vi "Create Fast Draw Object.vi"(6 "Actual Transform In":T1, 8 "error in (no error)":errorcluster, 9 "Multiplot Representation In":T3, 10 "3D Bar.lvclass in":refnum<class "3D Bar.lvclass">, 11 "Plot Object In":refnum<vi>) -> (0 "error out":errorcluster, 1 "Multiplot Representation Out":T3, 2 "3D Bar.lvclass out":refnum<class "3D Bar.lvclass">, 3 "Plot Object Out":refnum<vi>, 4 "Actual Transform Out":T1)   [LabVIEW 2017, in "3D Bar.lvclass"]
uses:
  <vilib>/Math Plots/3D Math Plots/3D Bar/3D Bar/3D Bar.lvclass
  <vilib>/Math Plots/3D Math Plots/3D Plot/3D Plot/Typedef/Multiplot Representation.ctl
  <vilib>/Math Plots/3D Math Plots/3D Plot/3D Plot/Typedef/Plot Representation.ctl
  <vilib>/Math Plots/3D Math Plots/3D Plot/3D Plot/Typedef/Range Clusters.ctl
  <vilib>/Math Plots/3D Math Plots/3D Plot/3D Plot/Typedef/Mesh Data.ctl
  <vilib>/Math Plots/3D Math Plots/3D Plot/3D Plot/Typedef/Actual Transform.ctl
  <vilib>/Math Plots/3D Math Plots/3D Bar/3D Bar/3D Bar.lvclass/3D Bar.ctl
  <vilib>/Math Plots/3D Math Plots/3D Plot/3D Plot/3D Plot.lvclass
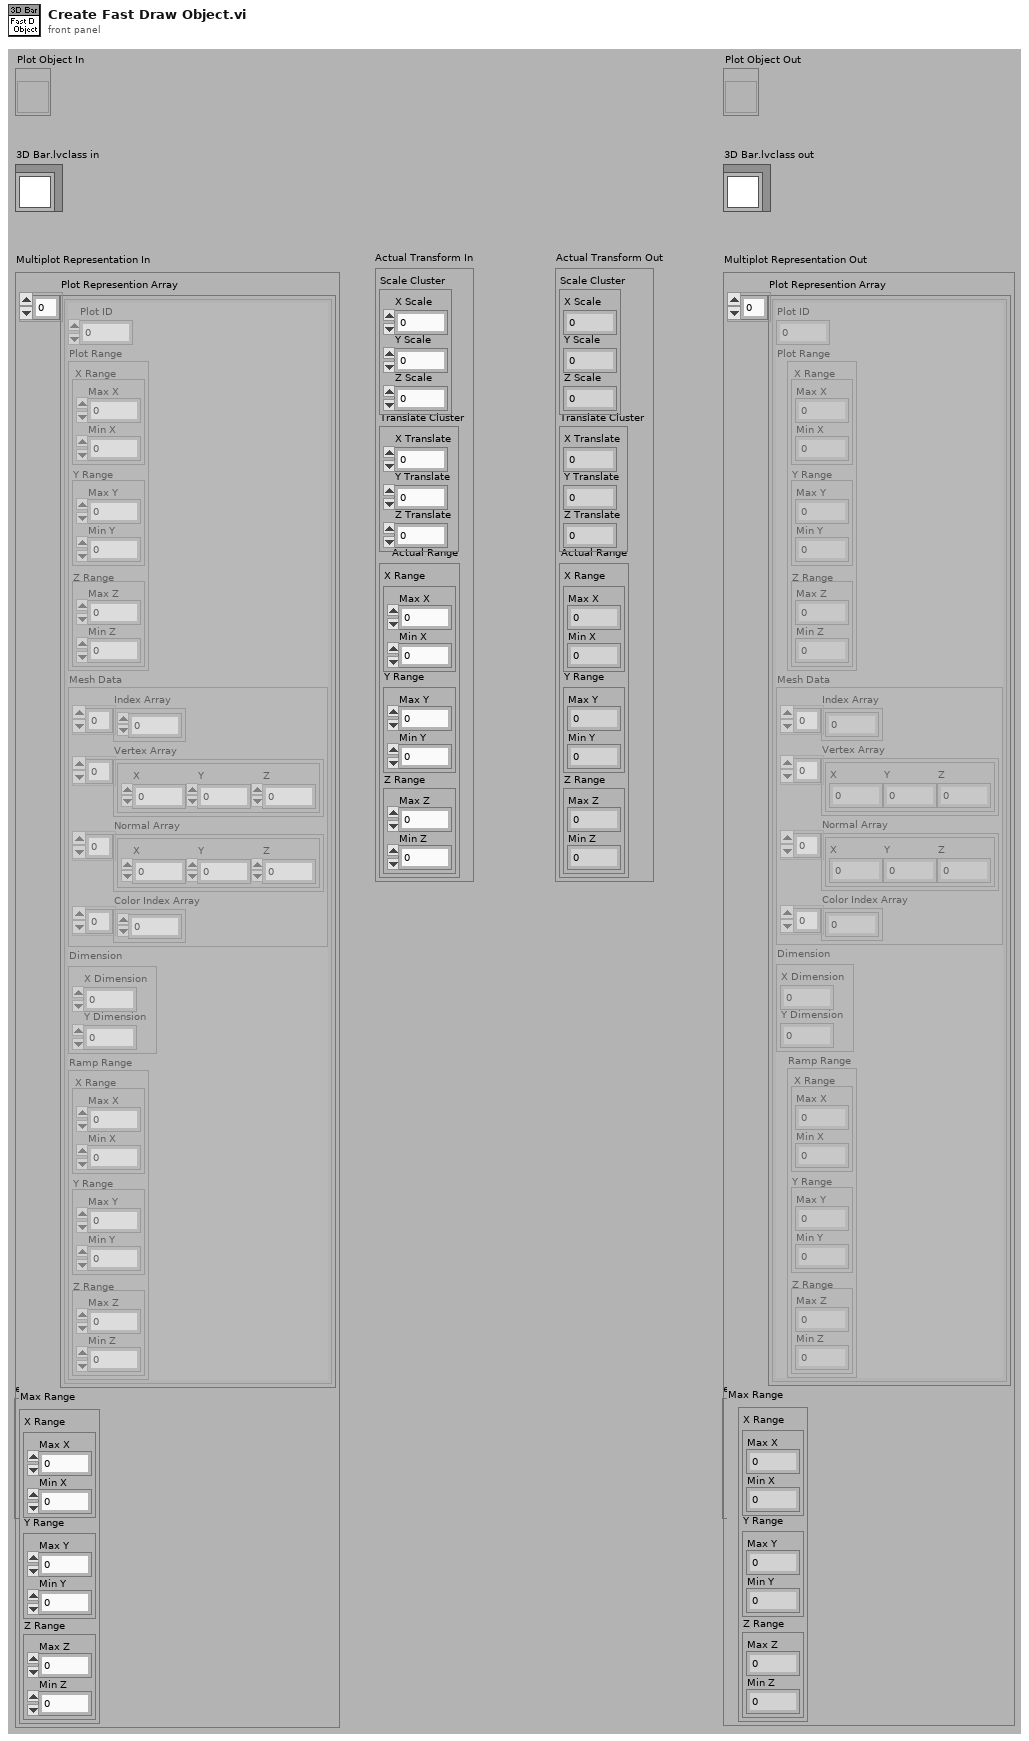
[diagram p1: front panel]
types:
  T1 = typedef "3D Plot.lvclass/Actual Transform.ctl" = cluster{"Scale Cluster":cluster{"X Scale":sgl, "Y Scale":sgl, "Z Scale":sgl}, "Translate Cluster":cluster{"X Translate":sgl, "Y Translate":sgl, "Z Translate":sgl}, "Actual Range":T2}
  T2 = typedef "3D Plot.lvclass/Range Clusters.ctl" = cluster{"X Range":cluster{"Max X":sgl, "Min X":sgl}, "Y Range":cluster{"Max Y":sgl, "Min Y":sgl}, "Z Range":cluster{"Max Z":sgl, "Min Z":sgl}}
  T3 = typedef "3D Plot.lvclass/Multiplot Representation.ctl" = cluster{"Plot Represention Array":T4[], "Max Range":T2}
  T4 = typedef "3D Plot.lvclass/Plot Representation.ctl" = cluster{"Plot ID":i32, "Plot Range":T2, "Mesh Data":T5, "Dimension":cluster{"X Dimension":i32, "Y Dimension":i32}, "Ramp Range":T2}
  T5 = typedef "3D Plot.lvclass/Mesh Data.ctl" = cluster{"Index Array":u32[], "Vertex Array":cluster{"X":sgl, "Y":sgl, "Z":sgl}[], "Normal Array":cluster{"X":sgl, "Y":sgl, "Z":sgl}[], "Color Index Array":i32[]}
  T6 = typedef "3D Bar.lvclass/3D Bar Property Array.ctl" = T7[]
  T7 = typedef "3D Bar.lvclass/3D Bar Property.ctl" = cluster{"General Property":cluster{"Plot Name":string, "Coordinate System":enum16{"Cartesian", "Cylindrical", "Spherical"}, "Opacity":sgl}, "Projection Property":cluster{"Draw XY":bool, "Draw YZ":bool, "Draw XZ":bool}, "Plot Property":cluster{"Line Style":T8, "Line Width":sgl, "Line Color":u32, "Antialiasing":bool}, "Bar Property":cluster{"Bar Mode":enum16{"Detach", "Group", "Stack"}, "Bar Width":sgl, "Color Pair Array":cluster{"Color":u32, "String":string}[]}}
  T8 = typedef "3D Plot.lvclass/Line Type.ctl" = enum16{"None", "Solid", "Dash", "Dot", "Dash Dot"}
  T9 = enum16{"Points", "Lines", "Line Strip", "Line Loop", "Triangles", "Triangle Strip", "Triangle Fan", "Quads", "Quad Strip", "Polygon"}
  T10 = cluster{"Draw XY":bool, "Draw YZ":bool, "Draw XZ":bool}
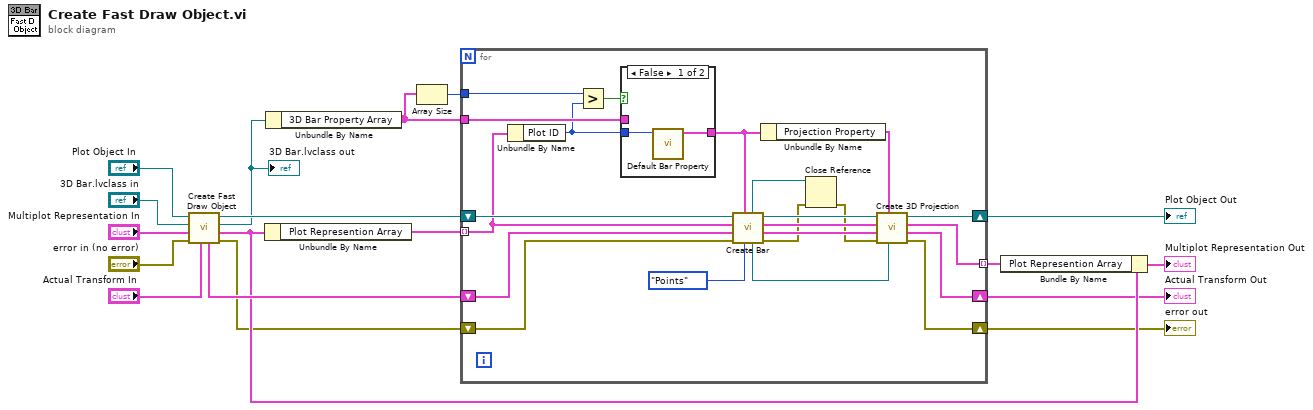
[diagram p0: block diagram]
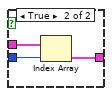
[diagram p2: hidden frame]
diagram:
  n1 = call-parent "Create Fast Draw Object.vi"("Actual Transform In"="Actual Transform In", "error in (no error)"="error in (no error)", "Multiplot Representation In"="Multiplot Representation In", "3D Plot.lvclass in"="3D Bar.lvclass in", "Plot Object In"="Plot Object In") -> ("error out"=w3:errorcluster, "Multiplot Representation Out"=w14:T3, "3D Plot.lvclass out"=w4:refnum<class "3D Bar.lvclass">, "Plot Object Out"=w16:refnum<vi>, "Actual Transform Out"=w15:T1)  [unwired: 2 out]
  "3D Bar.lvclass out" <- w4
  n2 = Unbundle By Name(w14) -> ("Plot Represention Array"=w18:T4[])
  n3 = Unbundle By Name(w4) -> ("3D Bar Property Array"=w1:T6)
  n4 = Array Size(array=w1) -> (size(s)=w2:i32)
  n5 = for {
    tunnel: w1 -> [w26]
    tunnel: w18 -> [w36] mode=indexing
    tunnel: [w37] -> w17 mode=indexing
    shift-right: [w34] -> w7
    shift-left: w15 -> [w28]
    shift-right: [w31] -> w5
    shift-left: w3 -> [w35]
    shift-right: [w32] -> w6
    shift-left: w16 -> [w38]
    tunnel: w2 -> [w23]
    n6 = Unbundle By Name(w36) -> ("Plot ID"=w24:i32)
    n7 = Greater?(x=w23, y=w24) -> (0:w27:bool)
    n8 = case shown="False" w27 {
      tunnel: w26 -> [_ w43]
      tunnel: [w39 w42] -> w25
      tunnel: w24 -> [w40 w41]
      frame False {
        n9 = call <vilib>:"Default Bar Property.vi"("Plot ID"=w40) -> ("Default Property"=w39:T7)  [unwired: 10 out]
      }
      frame True {
        n10 = Index Array(array=w43, index=w41) -> (element=w42:T7)
      }
    }
    n11 = call <vilib>:"Create Bar.vi"("Draw Mode"=T9."Points", "3D Bar Property"=w25, "error in (no error)"=w35, "Plot Representation In"=w36, "Plot Object In"=w38) -> ("error out"=w20:errorcluster, "Plot Representation Out"=w37:T4, "Plot Object Out"=w33:refnum<vi>, "Sector Object Out"=w30:refnum<vi>, "Bar Drawable"=w21:refnum<vi>)  [unwired: 1 in, 1 out]
    n12 = Unbundle By Name(w25) -> ("Projection Property"=w29:T10)
    n13 = Close Reference(reference=w21, error in (no error)=w20) -> (error out=w19:errorcluster)
    n14 = call <vilib>:"Create 3D Projection.vi"("Sub Object In"=w30, "Projection Property"=w29, "error in (no error)"=w19, "Actual Transform In"=w28, "Plot Object In"=w33) -> ("error out"=w31:errorcluster, "Actual Transform Out"=w34:T1, "Plot Object Out"=w32:refnum<vi>)  [unwired: 1 in, 3 out]
  }
  "error out" <- w5
  "Plot Object Out" <- w6
  "Actual Transform Out" <- w7
  n15 = Bundle By Name(cluster=w14, "Plot Represention Array"=w17) -> (→"Multiplot Representation Out":T3)
